vi "graph_waveform_arrays_activity_18.vi"() -> ()   [LabVIEW 2025]
panel:
  out "Waveform array":dbl[](array[numeric])
  out "Waveform Graph":dbl[][](graph)
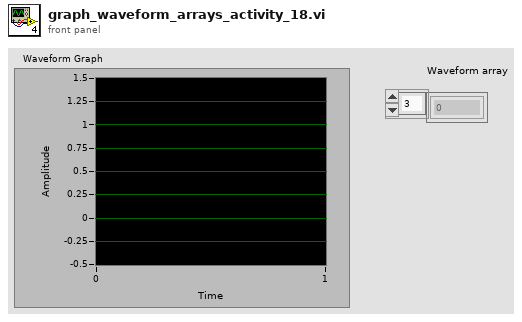
[diagram p1: front panel]
types:
  T1 = typedef "NI_Matrix.lvlib/RealMatrix.ctl" = dbl[][]
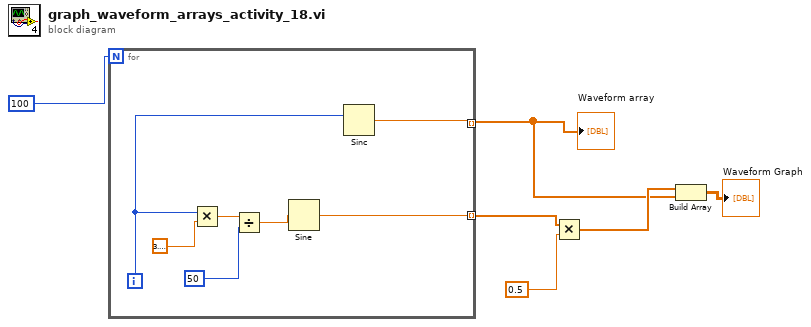
[diagram p0: block diagram]
diagram:
  n1 = for {
    N: 100 -> [_]
    tunnel: [w12] -> w2 mode=indexing
    tunnel: [w8] -> w4 mode=indexing
    i -> [w9]
    n2 = Multiply(x=w9, y=3.141592653589793) -> (x*y=w10:dbl)
    n3 = Divide(x=w10, y=50) -> (x/y=w13:dbl)
    n4 = Sine(x=w13) -> (sin(x)=w8:dbl)
    n5 = Sinc(1:w9) -> (0:w12:dbl)
  }
  "Waveform array" <- w2
  n6 = Multiply(x=w4, y=0.5) -> (x*y=w3:dbl[])
  n7 = Build Array(w3, w2) -> (→"Waveform Graph":T1)
